vi "StanfordVoltage.vi"() -> ()   [LabVIEW 2013]
panel:
  out "Stanford Voltage":dbl
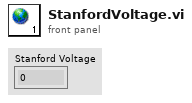
[diagram p1: front panel]
diagram:
